vi "Script_Excit_Extract_Values_From_Wfm_Name.vi"(8 "error in (no error)":errorcluster, 11 "Excit Wfm String":string="E1TwoSwift0p5f250p0to600p0a70and700p0to1000p0a50d1200fs10") -> (0 "error out":errorcluster, 3 "Excit Wfm Values":string[](array[string]))   [LabVIEW 2017]
uses:
  controls/EXCIT_Form_Selector.ctl
panel:
  in  "Excit Form":T1=enum."TwoSwift"
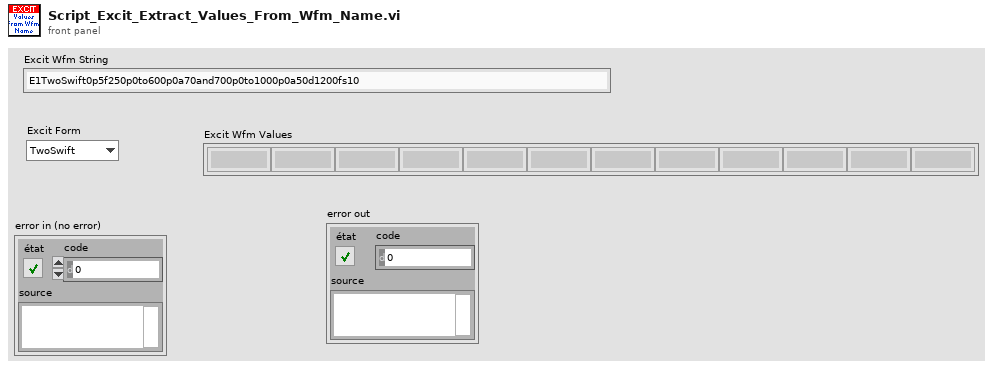
[diagram p1: front panel]
types:
  T1 = typedef "EXCIT_Form_Selector.ctl" = enum16{"Swift", "TwoSwift", "Chirp", "Sinus", "Ramp"}
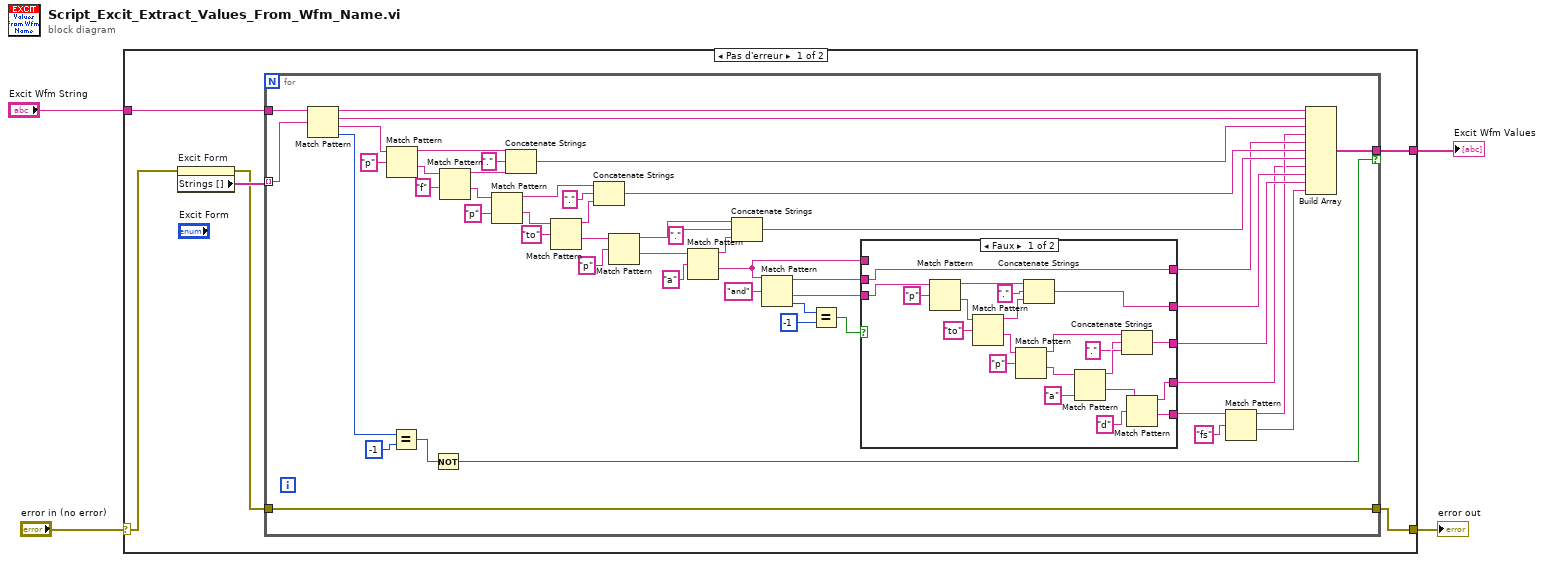
[diagram p0: block diagram]
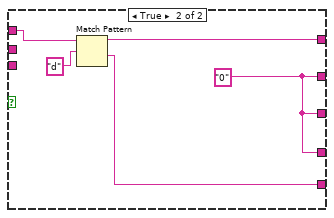
[diagram p2: hidden frame]
diagram:
  n1 = case shown="Pas d'erreur" "error in (no error)" {
    selector: "error in (no error)" -> [w7 w86]
    tunnel: [w10 _] -> w4
    tunnel: "Excit Wfm String" -> [w9 _]
    tunnel: [w5 w86] -> w1
    frame No Error {
      n2 = property on="Excit Form" class="Énum (strict)"(error in=w7) -> (error out=w6:errorcluster, "Strings []"=w8:string[])  [unwired: 1 in, 1 out]
      n3 = for {
        tunnel: w8 -> [w59] mode=indexing
        tunnel: w9 -> [w15]
        tunnel: [w16] -> w10 if=w25
        tunnel: w6 -> [w11]
        tunnel: [w11] -> w5
        n4 = Match Pattern(string=w15, regular expression=w59) -> (before substring=w24:string, match substring=w23:string, after substring=w55:string, offset past match=w58:i32)  [unwired: 1 in]
        n5 = Match Pattern(string=w55, regular expression="p" ("expression régulière")) -> (before substring=w51:string, after substring=w53:string)  [unwired: 1 in, 2 out]
        n6 = Equal?(x=w58, y=-1) -> (x = y?=w56:bool)
        n7 = Not(x=w56) -> (.not. x?=w25:bool)
        n8 = Match Pattern(string=w53, regular expression="f" ("expression régulière")) -> (before substring=w50:string, after substring=w48:string)  [unwired: 1 in, 2 out]
        n9 = Match Pattern(string=w48, regular expression="p" ("expression régulière")) -> (before substring=w45:string, after substring=w44:string)  [unwired: 1 in, 2 out]
        n10 = Concatenate Strings(w51, "." ("chaîne"), w50) -> (w22:string)
        n11 = Match Pattern(string=w44, regular expression="to" ("expression régulière")) -> (before substring=w42:string, after substring=w41:string)  [unwired: 1 in, 2 out]
        n12 = Concatenate Strings(w45, "." ("chaîne"), w42) -> (w21:string)
        n13 = Match Pattern(string=w41, regular expression="p" ("expression régulière")) -> (before substring=w39:string, after substring=w37:string)  [unwired: 1 in, 2 out]
        n14 = Match Pattern(string=w37, regular expression="a" ("expression régulière")) -> (before substring=w35:string, after substring=w29:string)  [unwired: 1 in, 2 out]
        n15 = Concatenate Strings(w39, "." ("chaîne"), w35) -> (w20:string)
        n16 = Match Pattern(string=w29, regular expression="and" ("expression régulière")) -> (before substring=w27:string, after substring=w26:string, offset past match=w32:i32)  [unwired: 1 in, 1 out]
        n17 = Equal?(x=w32, y=-1) -> (x = y?=w30:bool)
        n18 = case shown="Faux" w30 {
          tunnel: w29 -> [_ w85]
          tunnel: [w78 w82] -> w14
          tunnel: [w79 w83] -> w28
          tunnel: [w68 w81] -> w19
          tunnel: [w61 w81] -> w18
          tunnel: [w60 w81] -> w12
          tunnel: w27 -> [w78 _]
          tunnel: w26 -> [w77 _]
          frame False {
            n19 = Match Pattern(string=w77, regular expression="p" ("expression régulière")) -> (before substring=w71:string, after substring=w75:string)  [unwired: 1 in, 2 out]
            n20 = Match Pattern(string=w75, regular expression="to" ("expression régulière")) -> (before substring=w69:string, after substring=w73:string)  [unwired: 1 in, 2 out]
            n21 = Match Pattern(string=w73, regular expression="p" ("expression régulière")) -> (before substring=w62:string, after substring=w66:string)  [unwired: 1 in, 2 out]
            n22 = Concatenate Strings(w71, "." ("chaîne"), w69) -> (w68:string)
            n23 = Match Pattern(string=w66, regular expression="a" ("expression régulière")) -> (before substring=w64:string, after substring=w67:string)  [unwired: 1 in, 2 out]
            n24 = Concatenate Strings(w62, "." ("chaîne"), w64) -> (w61:string)
            n25 = Match Pattern(string=w67, regular expression="d" ("expression régulière")) -> (before substring=w60:string, after substring=w79:string)  [unwired: 1 in, 2 out]
          }
          frame True {
            w81 = "0"
            n26 = Match Pattern(string=w85, regular expression="d" ("expression régulière")) -> (before substring=w82:string, after substring=w83:string)  [unwired: 1 in, 2 out]
          }
        }
        n27 = Match Pattern(string=w28, regular expression="fs" ("expression régulière")) -> (before substring=w13:string, after substring=w17:string)  [unwired: 1 in, 2 out]
        n28 = Build Array(w24, w23, w22, w13, w14, w21, w20, w12, w19, w18, w17) -> (w16:string[])
      }
    }
    frame Error {
    }
  }
  "Excit Wfm Values" <- w4
  "error out" <- w1
